vi "Force_sensor_file.vi"(7 "cmd":enum16{"Sensor file create", "Sensor file read"}(ring)=enum."Sensor file read", 8 "error in":errorcluster, 10 "file path":path, 11 "Force Sensor data in":T1) -> (0 "error out":errorcluster, 3 "Force Sensor data out":T1)   [LabVIEW 2016]
uses:
  ctl/force_sensor_data.ctl
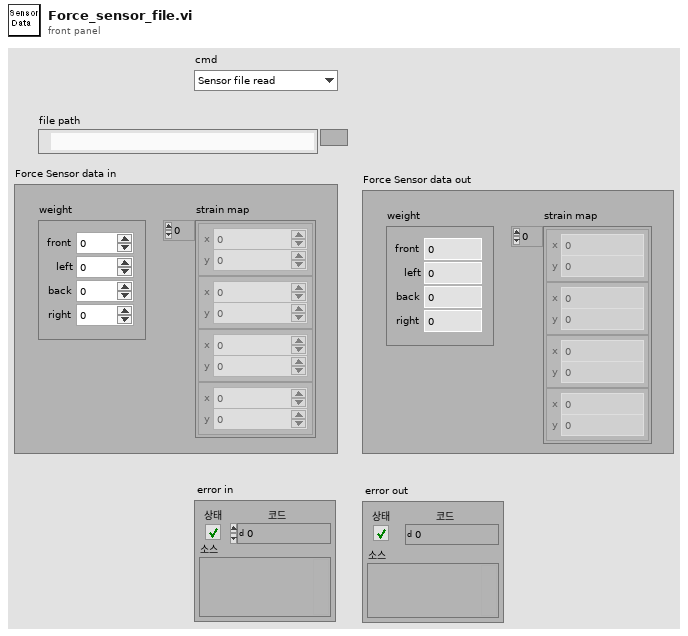
[diagram p1: front panel]
types:
  T1 = typedef "force_sensor_data.ctl" = cluster{"weight":cluster{"front":dbl, "left":dbl, "back":dbl, "right":dbl}, "strain map":cluster{"x":dbl, "y":dbl}[]}
  T2 = enum16{"open", "replace", "create", "open or create", "replace or create", "replace or create with confirmation"}
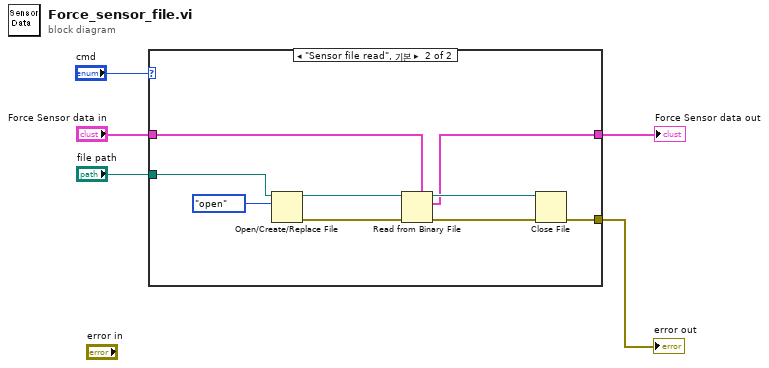
[diagram p0: block diagram]
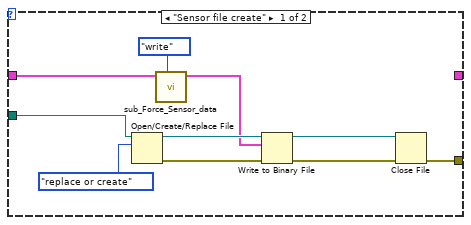
[diagram p2: hidden frame]
diagram:
  n1 = case shown="\"Sensor file read\", 기본" "cmd" {
    tunnel: [_ w19] -> w4
    tunnel: "Force Sensor data in" -> [w8 w18]
    tunnel: [w7 w17] -> w2
    tunnel: "file path" -> [w6 w16]
    frame "Sensor file create" {
      n2 = Open/Create/Replace File(file path (use dialog)=w6, operation (0:open)=T2."replace or create" ("동작(0:open)")) -> (refnum out=w12:refnum<file>, error out=w15:errorcluster)  [unwired: 4 in, 1 out]
      n3 = call "sub_Force_Sensor_data.vi"("cmd"=enum16{"write", "read"}."write", "Force Sensor data"=w8) -> ("Force Sensor data out"=w9:T1)  [unwired: 9 in]
      n4 = Write to Binary File(file (use dialog)=w12, data=w9, error in=w15) -> (refnum out=w13:refnum<file>, error out=w14:errorcluster)  [unwired: 3 in, 1 out]
      n5 = Close File(refnum=w13, error in=w14) -> (error out=w7:errorcluster)  [unwired: 1 out]
    }
    frame "Sensor file read", Default {
      n6 = Open/Create/Replace File(file path (use dialog)=w16, operation (0:open)=T2."open" ("동작(0:open)")) -> (refnum out=w21:refnum<file>, error out=w24:errorcluster)  [unwired: 4 in, 1 out]
      n7 = Read from Binary File(5:w18, 8:w24, 11:w21) -> (0:w23:errorcluster, 2:w19:T1, 3:w22:refnum<file>)  [unwired: 3 in, 1 out]
      n8 = Close File(refnum=w22, error in=w23) -> (error out=w17:errorcluster)  [unwired: 1 out]
    }
  }
  "Force Sensor data out" <- w4
  "error out" <- w2
